vi "Configure Measurement (Period).vi"(7 "Frequency Resolution (100E-9s)":dbl=1e-07 format="%^#_7g", 8 "error in (no error)":errorcluster, 9 "Period Estimate (100E-9s)":dbl=1e-07 format="%^#_7g", 10 "Channel (1:Channel 1)":i32(ring)=1 items=["Channel 1"=1, "Channel 2"=2], 11 "VISA resource name":refnum<visa-resource-name>) -> (0 "error out":errorcluster, 3 "VISA resource name out":refnum<visa-resource-name>)   [LabVIEW 2020, in "Template - Counter.lvlib"]
doc: "Configures the parameters required for Period measurements."
uses:
  <instrlib>/_Template - Counter/Template - Counter.lvlib
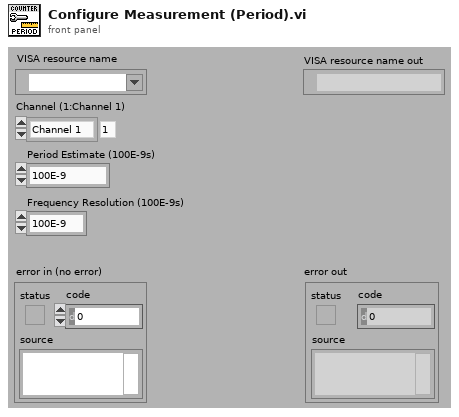
[diagram p1: front panel]
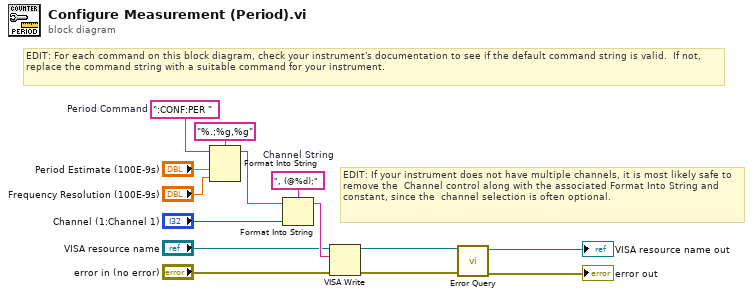
[diagram p0: block diagram]
diagram:
  w13 = ", (@%d);"  # Channel String
  w2 = ":CONF:PER "  # Period Command
  # "EDIT: If your instrument does not have multiple channels, it is most likely safe to remove the  Channel control along with the associated Format Into String and constant, since the  channel selection is often optional."
  # "EDIT: For each command on this block diagram, check your instrument's documentation to see if the default command string is valid.  If not, replace the command string with a suitable command for your instrument."
  n1 = Format Into String(format string="%.;%g,%g", initial string=w2, "Period Estimate (100E-9s)", "Frequency Resolution (100E-9s)") -> (resulting string=w3:string)  [unwired: 1 in, 1 out]
  n2 = Format Into String(format string=w13, initial string=w3, "Channel (1:Channel 1)") -> (resulting string=w10:string)  [unwired: 1 in, 1 out]
  n3 = VISA Write(VISA resource name="VISA resource name", write buffer=w10, error in (no error)="error in (no error)") -> (VISA resource name out=w12:refnum<visa-resource-name>, error out=w11:errorcluster)  [unwired: 1 out]
  n4 = call <instrlib>:"Error Query.vi"("error in (no error)"=w11, "VISA resource name"=w12) -> ("error out"=→"error out":errorcluster, "VISA resource name out"=→"VISA resource name out":refnum<visa-resource-name>)  [unwired: 6 in, 2 out]
